vi "Init Size.vi"(8 "error in (no error)":errorcluster, 10 "Size":u32, 11 "Vector Parent in":refnum<class "Vector Parent.lvclass">) -> (0 "error out":errorcluster, 3 "Vector Parent out":refnum<class "Vector Parent.lvclass">)   [LabVIEW 2021, in "Vector Parent.lvclass"]
uses:
  Vector Parent.lvclass
  Vector Parent.lvclass/Vector Parent.ctl
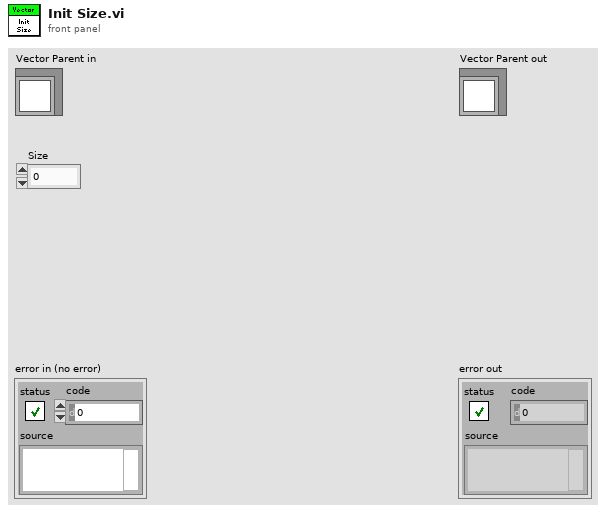
[diagram p1: front panel]
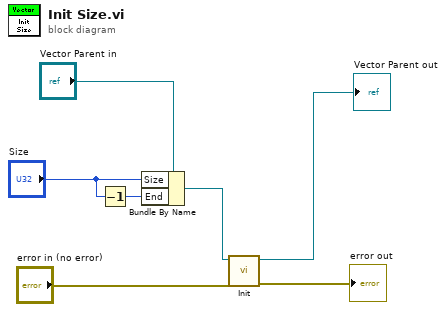
[diagram p0: block diagram]
diagram:
  n1 = Decrement(x="Size") -> (x-1=w5:u32)
  n2 = Bundle By Name(cluster="Vector Parent in", "Size"="Size", "End"=w5) -> (w2:refnum<class "Vector Parent.lvclass">)
  n3 = call-dynamic "Init.vi"("error in (no error)"="error in (no error)", "Data in"=w2) -> ("error out"=→"error out":errorcluster, "Data out"=→"Vector Parent out":refnum<class "Vector Parent.lvclass">)  [unwired: 8 in]
